vi "Measurement Logic.vi"() -> ()   [LabVIEW 2021, in "Line Transient Response_PMIC.lvlib"]
uses:
  Line Transient Response_PMIC.lvlib
  <vilib>/Plug-In SDKs/Measurements/Measure Call Context/Measure Call Context.lvclass
  Measurement Results.ctl
  Measurement Configuration.ctl
  <instrlib>/niDCPower/nidcpower.llb/niDCPower Source Mode.ctl
  <instrlib>/niDCPower/nidcpower.llb/niDCPower Wait For Event - Event.ctl
  <instrlib>/niScope/Controls/niScope trigger slope.ctl
  <instrlib>/niDCPower/nidcpower.llb/niDCPower Output Function.ctl
  <instrlib>/niDCPower/nidcpower.llb/niDCPower Aperture Time Units.ctl
  <instrlib>/niDCPower/nidcpower.llb/niDCPower Get Channel Name From String.vi
  <instrlib>/niScope/Utility/niScope Get Channel Name From String.vi
  <instrlib>/niScope/Configure/Trigger/niScope Configure Trigger Digital.vi
  <instrlib>/niDCPower/nidcpower.llb/niDCPower Configure Digital Edge Measure Trigger With Channels.vi
  <instrlib>/niDCPower/nidcpower.llb/niDCPower Configure Digital Edge Source Trigger With Channels.vi
  <instrlib>/niScope/Acquire/Fetch/niScope Fetch.vi
panel:
  in  "measurement configuration":T1={"DUT setup time"=1.0, "Nominal output voltage"=3.3, "Source resource name"="", "Source current limit"=0.25, "Source maximum power"=300.0, "Source sample rate"=1800000.0, "Source voltage set point 1"=7.0, "Source voltage set point 2"=20.0, "Source voltatge pulse duration"=0.005, "Source voltage delay t1"=0.005, "Source voltage delay t2"=0.005, "Source voltage falling slew rate"=50000.0, "Source voltage rising slew rate"=50000.0, "Source transient response"=1042, "Source voltage gain bandwidth"=2000.0, "Source voltage compensation frequency"=3530.0, "Source voltage pole-zero ratio"=2.0, "Load resource name"="", "Load voltage limit range"=4.0, "Load current level range"=4.0, "Load current level"=0.03, "Load transient response"=1042, "Load current gain bandwidth"=14000.0, "Load current compensation frequency"=180000.0, "Load current pole-zero ratio"=0.3, "Scope resource name"="", "Scope enable/disable"=TRUE, "Scope output channel name"="0", "Scope sample rate"=1800000.0, "Scope probe attenuation"=1.0, "Scope vertical range"=10.0, "Scope vertical coupling"=enum."DC", "Source Sense"=1008, "Load Sense"=1009, "Source update rate"=1000.0} {"Source update rate" format="%#_6pS/s"; "Load Sense" items=["Local"=1008, "Remote"=1009]; "Source Sense" items=["Local"=1008, "Remote"=1009]; "Source voltage delay t1" format="%#_8g"; "Scope vertical range" format="%.2f"; "Scope probe attenuation" format="%.1f"; "Scope sample rate" step=1000000.0 format="%#.2g"; "Load transient response" items=["Slow"=1041, "Normal"=1038, "Fast"=1039, "Custom"=1042]; "Source transient response" items=["Slow"=1041, "Normal"=1038, "Fast"=1039, "Custom"=1042]}
  out "measurement results":T2
  out "measure call context out":refnum<class "Measure Call Context.lvclass">
  in  "measure call context in":refnum<class "Measure Call Context.lvclass">
  out "error out":errorcluster
  in  "error in":errorcluster
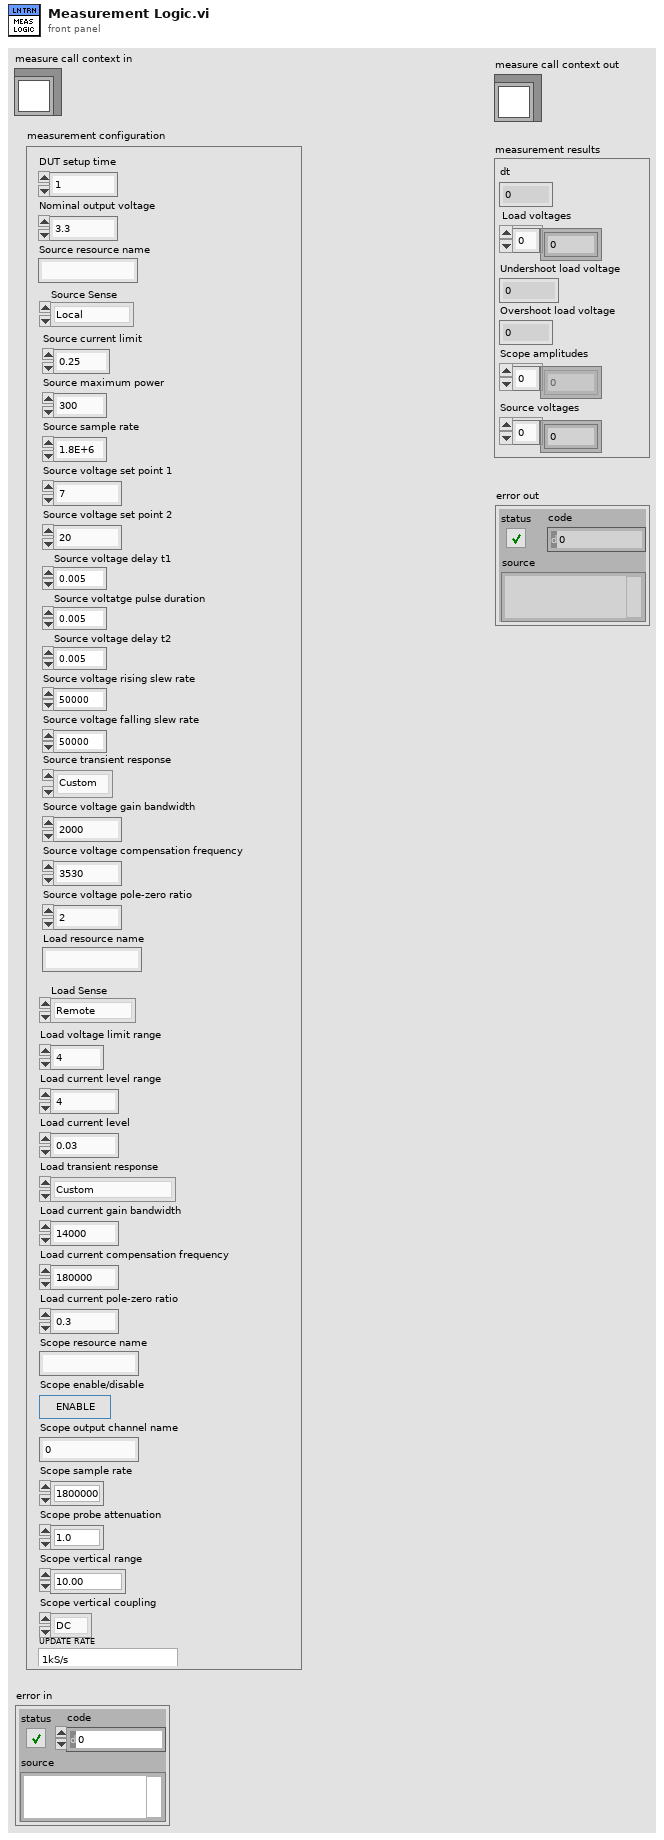
[diagram p1: front panel]
types:
  T1 = typedef "Line Transient Response_PMIC.lvlib/Measurement Configuration.ctl" = cluster{"DUT setup time":dbl, "Nominal output voltage":dbl, "Source resource name":string, "Source current limit":dbl, "Source maximum power":dbl, "Source sample rate":dbl, "Source voltage set point 1":dbl, "Source voltage set point 2":dbl, "Source voltatge pulse duration":dbl, "Source voltage delay t1":dbl, "Source voltage delay t2":dbl, "Source voltage falling slew rate":dbl, "Source voltage rising slew rate":dbl, "Source transient response":i32, "Source voltage gain bandwidth":dbl, "Source voltage compensation frequency":dbl, "Source voltage pole-zero ratio":dbl, "Load resource name":string, "Load voltage limit range":dbl, "Load current level range":dbl, "Load current level":dbl, "Load transient response":i32, "Load current gain bandwidth":dbl, "Load current compensation frequency":dbl, "Load current pole-zero ratio":dbl, "Scope resource name":string, "Scope enable/disable":bool, "Scope output channel name":string, "Scope sample rate":dbl, "Scope probe attenuation":dbl, "Scope vertical range":dbl, "Scope vertical coupling":enum32{"AC", "DC"}, "Source Sense":i32, "Load Sense":i32, "Source update rate":dbl}
  T2 = typedef "Line Transient Response_PMIC.lvlib/Measurement Results.ctl" = cluster{"dt":dbl, "Load voltages":dbl[], "Undershoot load voltage":dbl, "Overshoot load voltage":dbl, "Scope amplitudes":dbl[], "Source voltages":dbl[]}
  T3 = cluster{"Source out":refnum<k15>, "Source channel name":string, "Load out":refnum<k15>, "Load channel name":string, "Scope out":refnum<k15>, "Scope channel name":string, "Source sequence name":string, "Source terminal name":string, "Start source terminal name":string, "Measure load and scope terminal name":string, "Measure record length smu":i32, "Aperture time":dbl, "Measure record length scope":i32, "measurement results":T2}
  T4 = typedef "niDCPower Wait For Event - Event.ctl" = i32
  T5 = typedef "niDCPower Source Mode.ctl" = i32
  T6 = typedef "niScope trigger slope.ctl" = i32
  T7 = typedef "niDCPower Aperture Time Units.ctl" = i32
  T8 = typedef "niDCPower Output Function.ctl" = i32
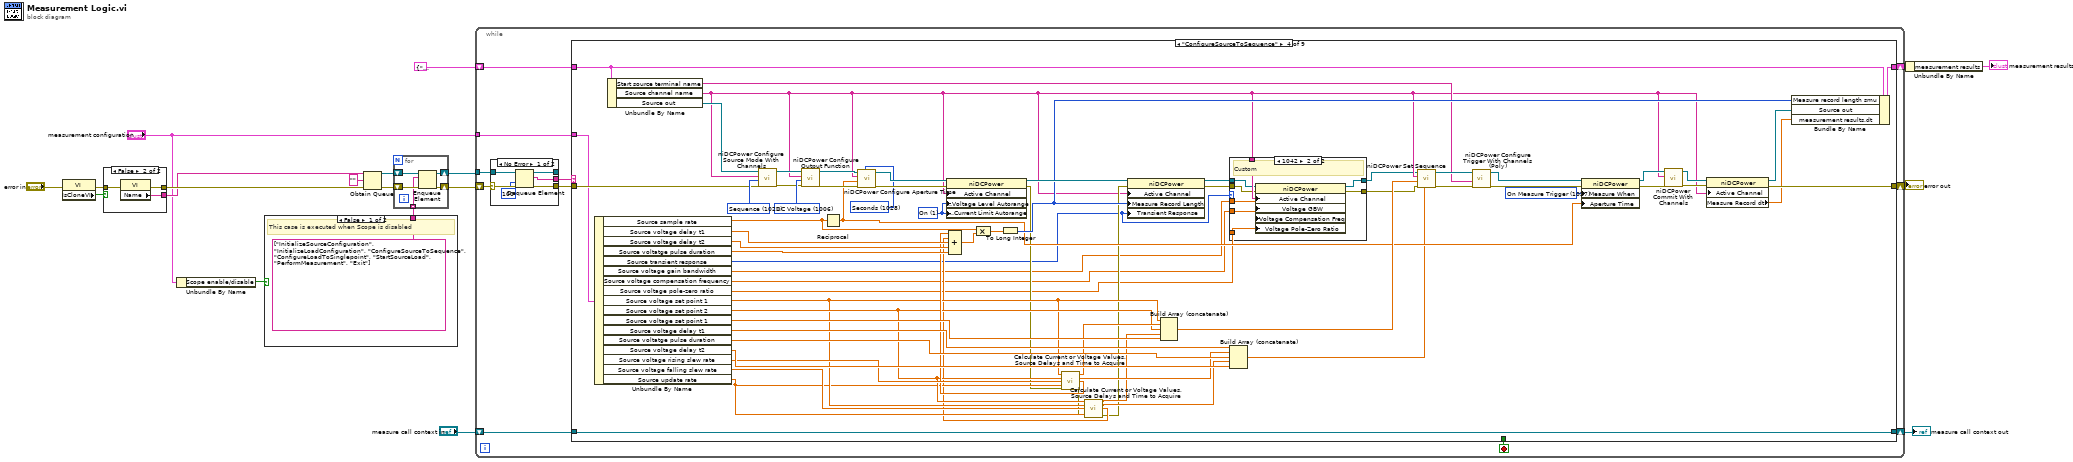
[diagram p0: block diagram]
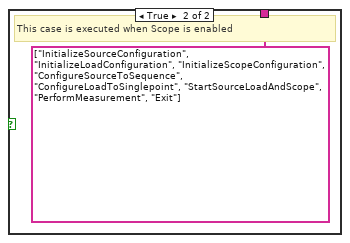
[diagram p2: hidden frame]
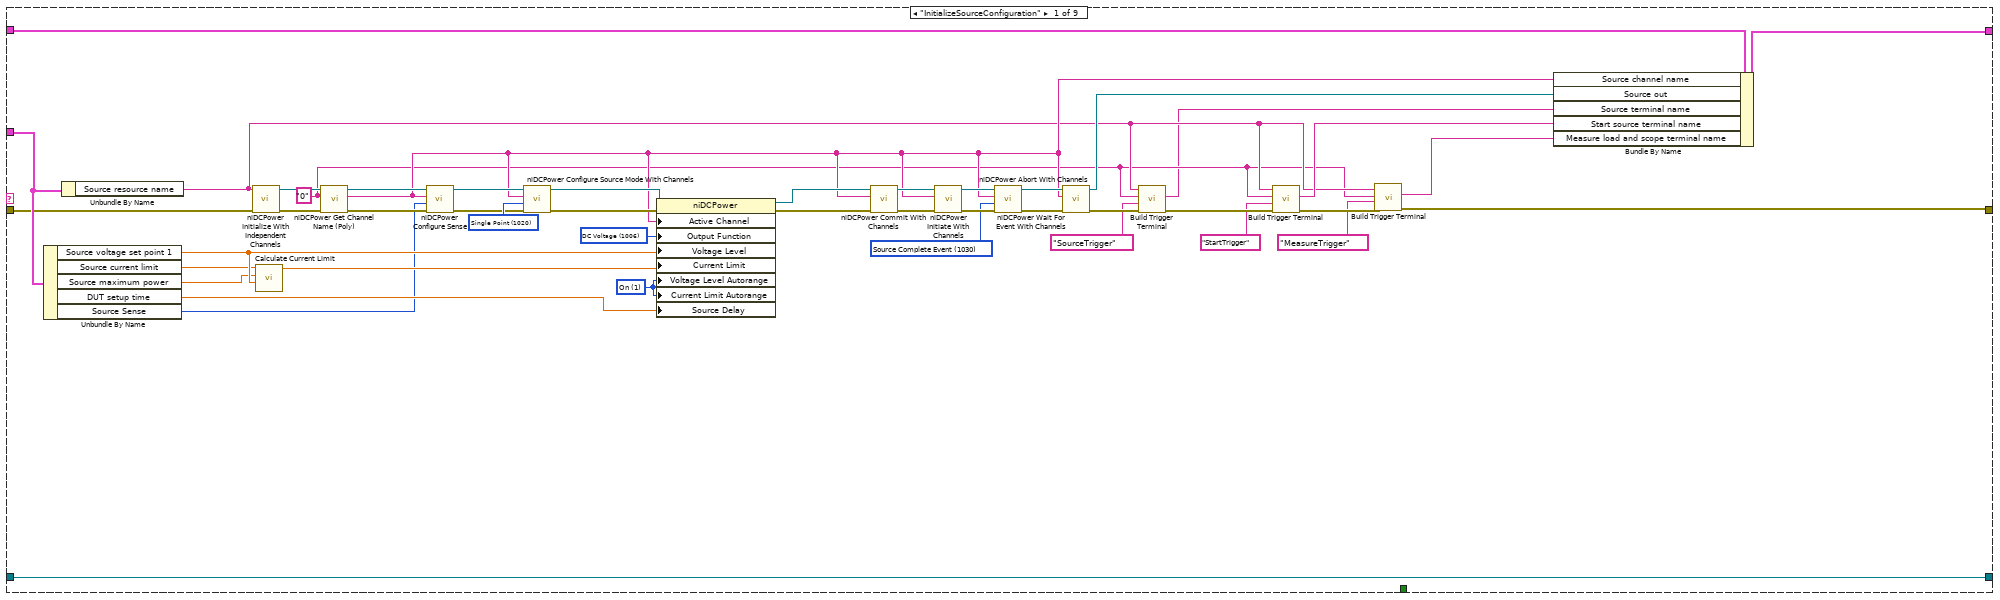
[diagram p3: hidden frame]
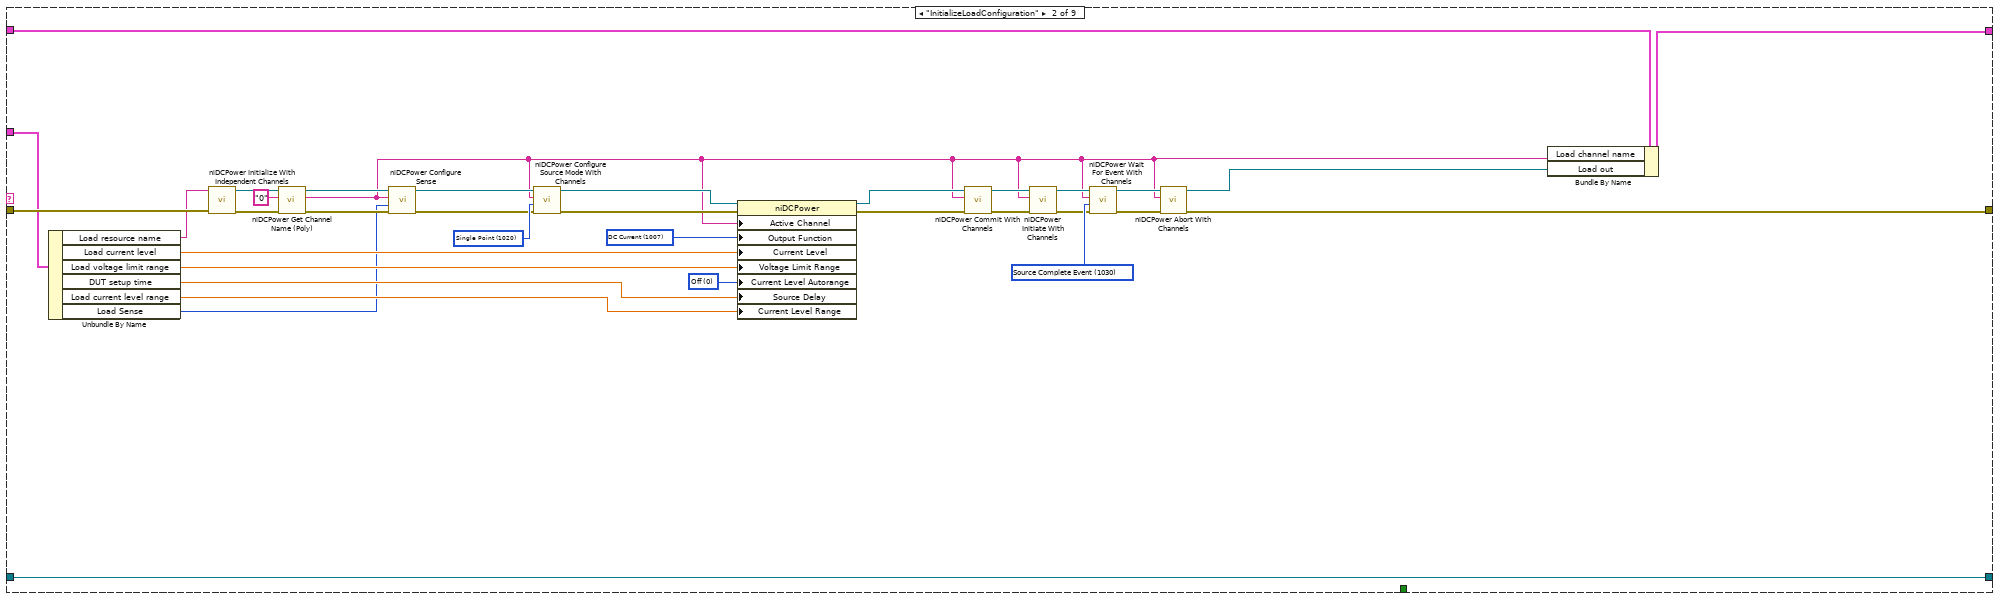
[diagram p4: hidden frame]
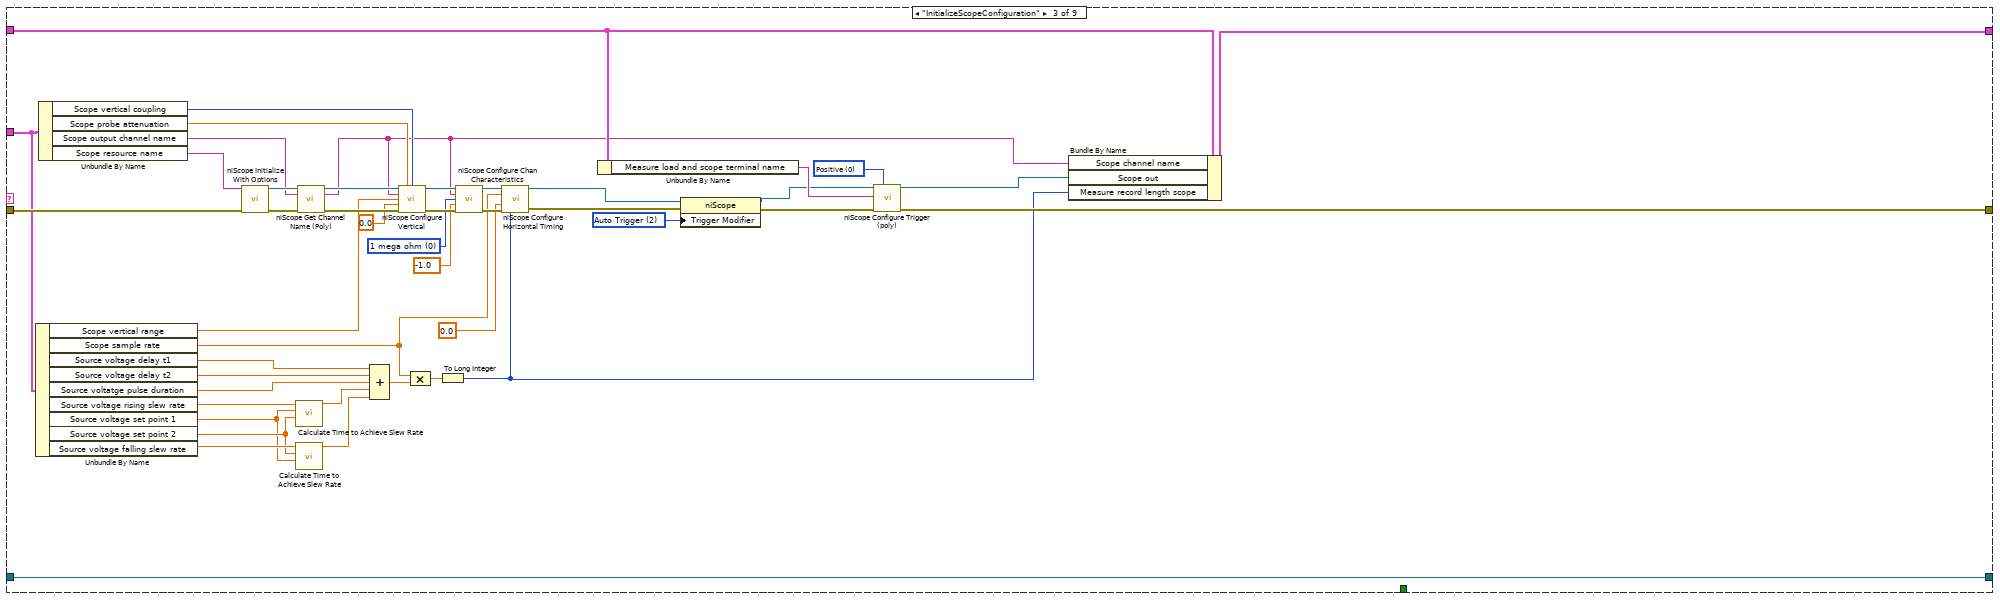
[diagram p5: hidden frame]
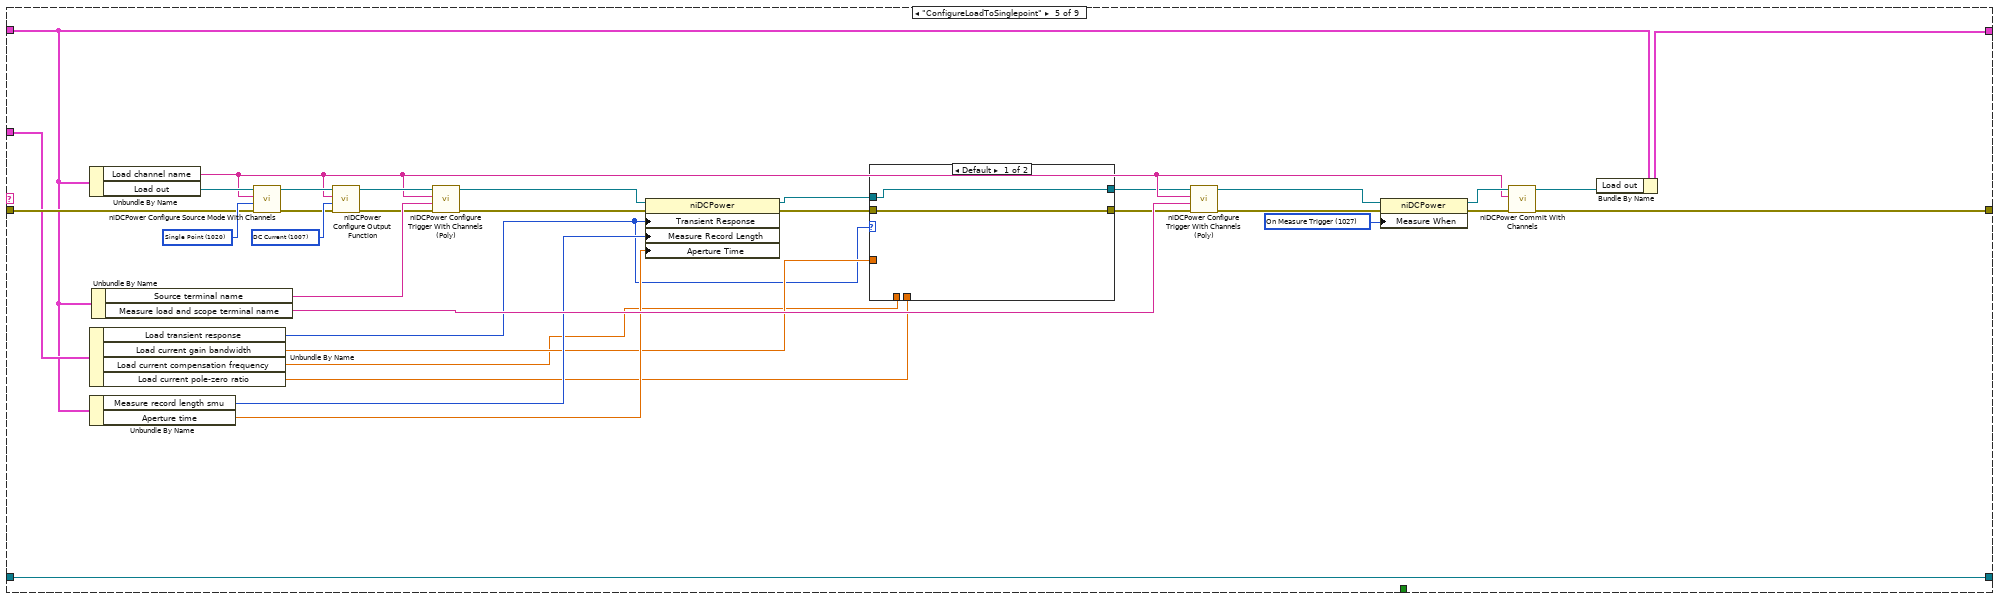
[diagram p7: hidden frame]
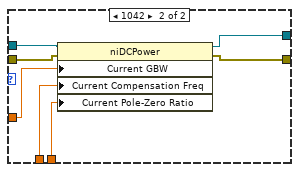
[diagram p8: hidden frame]
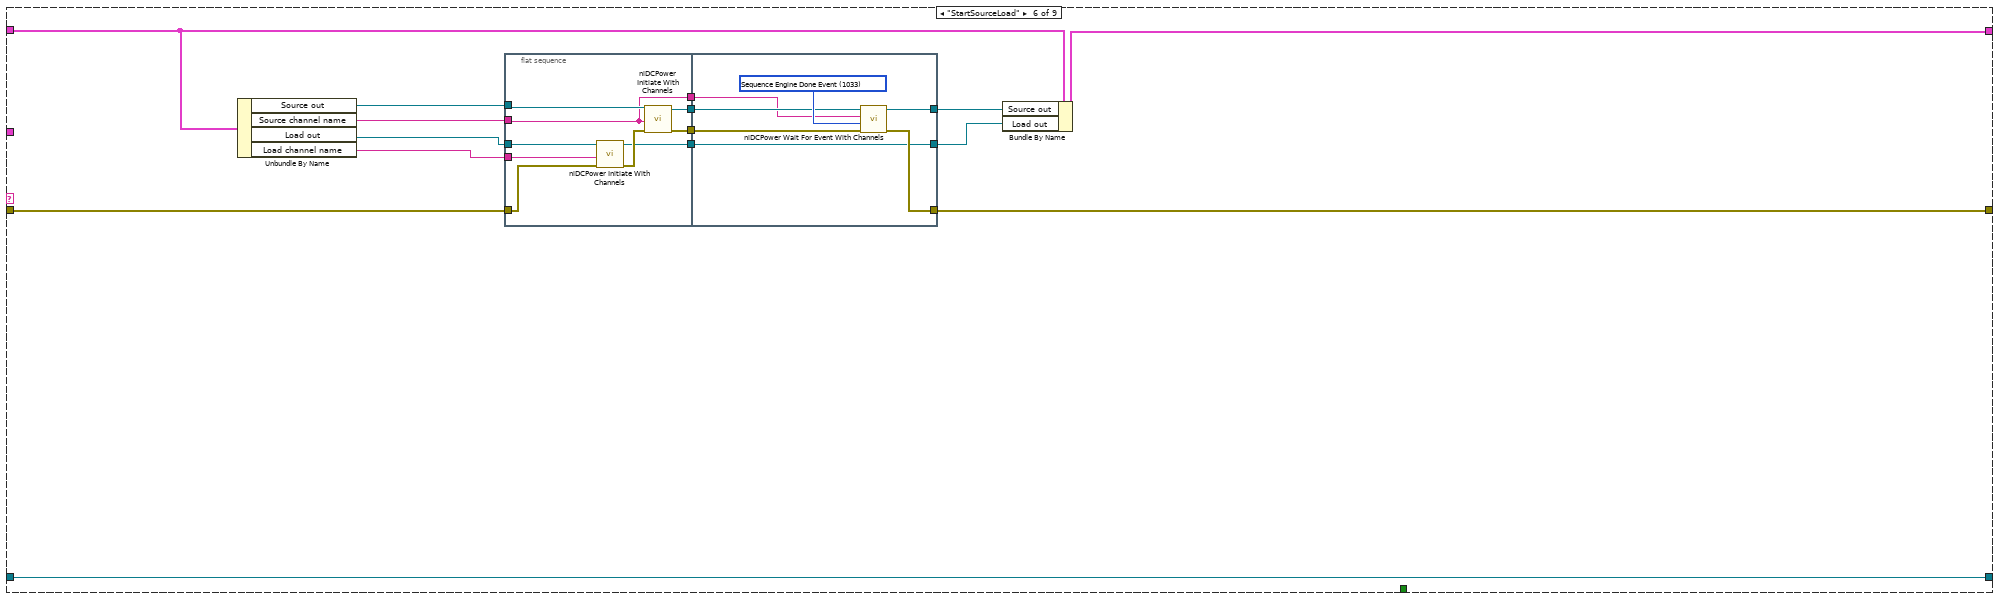
[diagram p9: hidden frame]
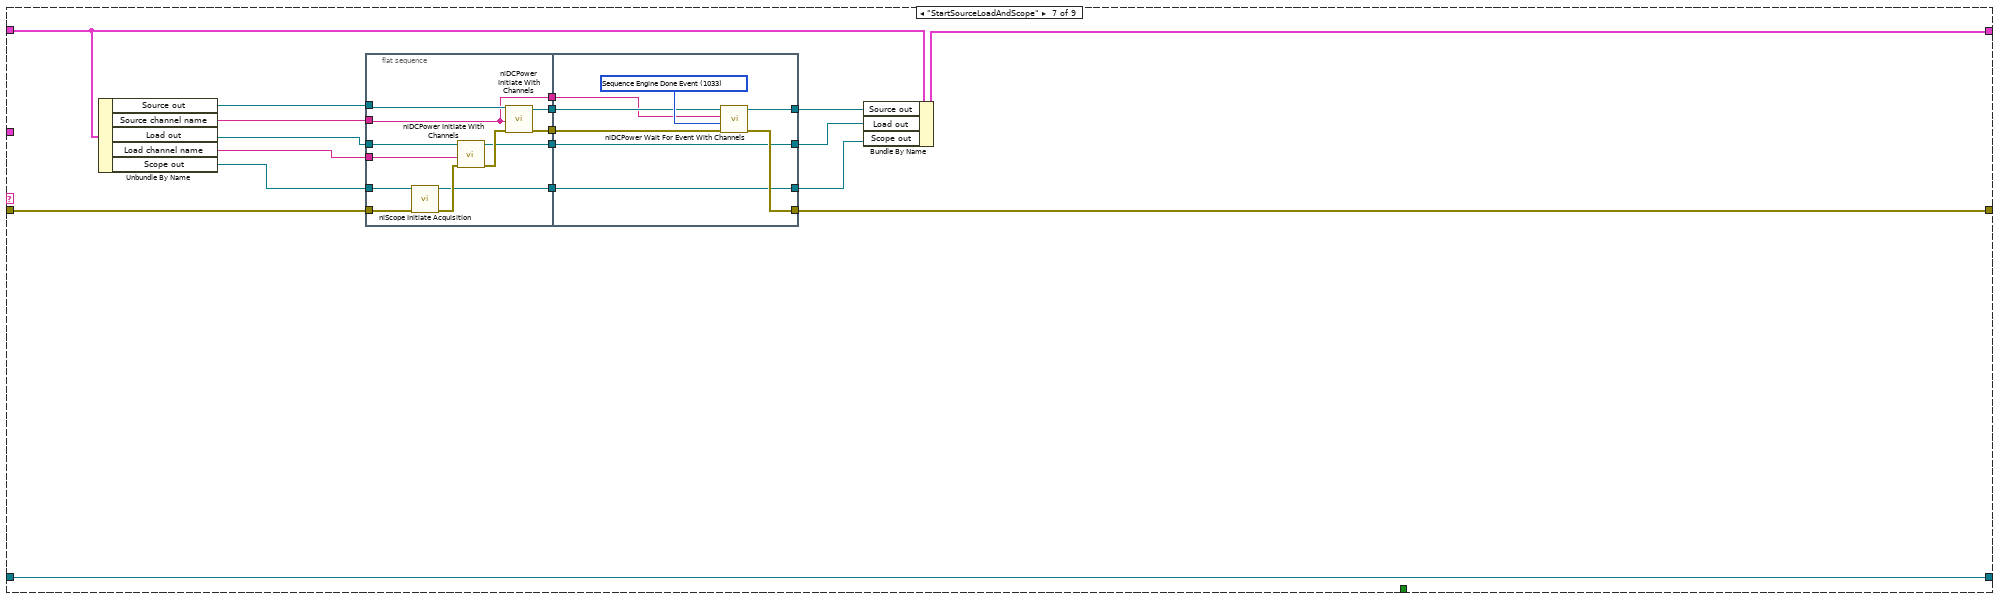
[diagram p10: hidden frame]
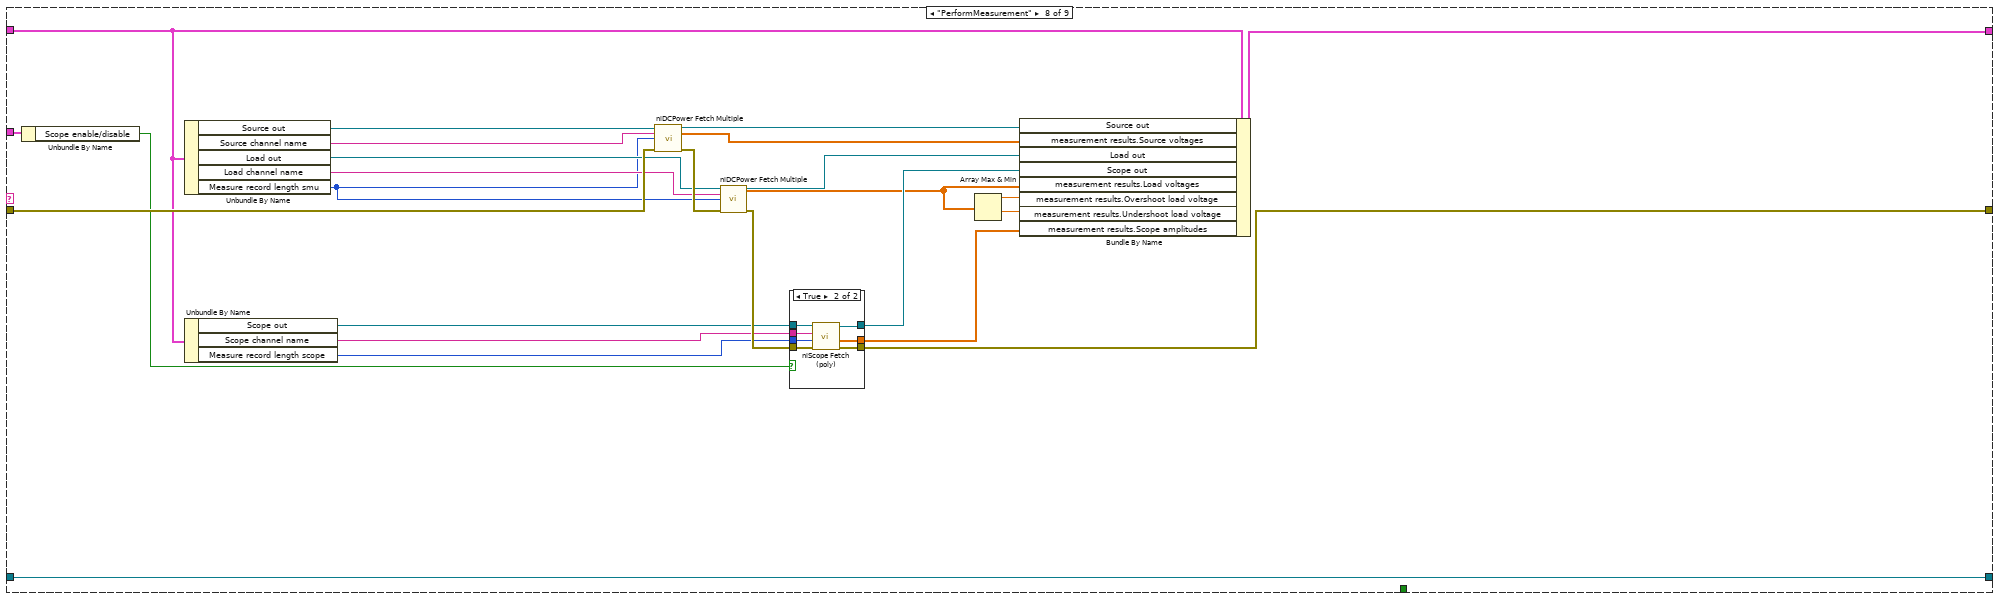
[diagram p11: hidden frame]
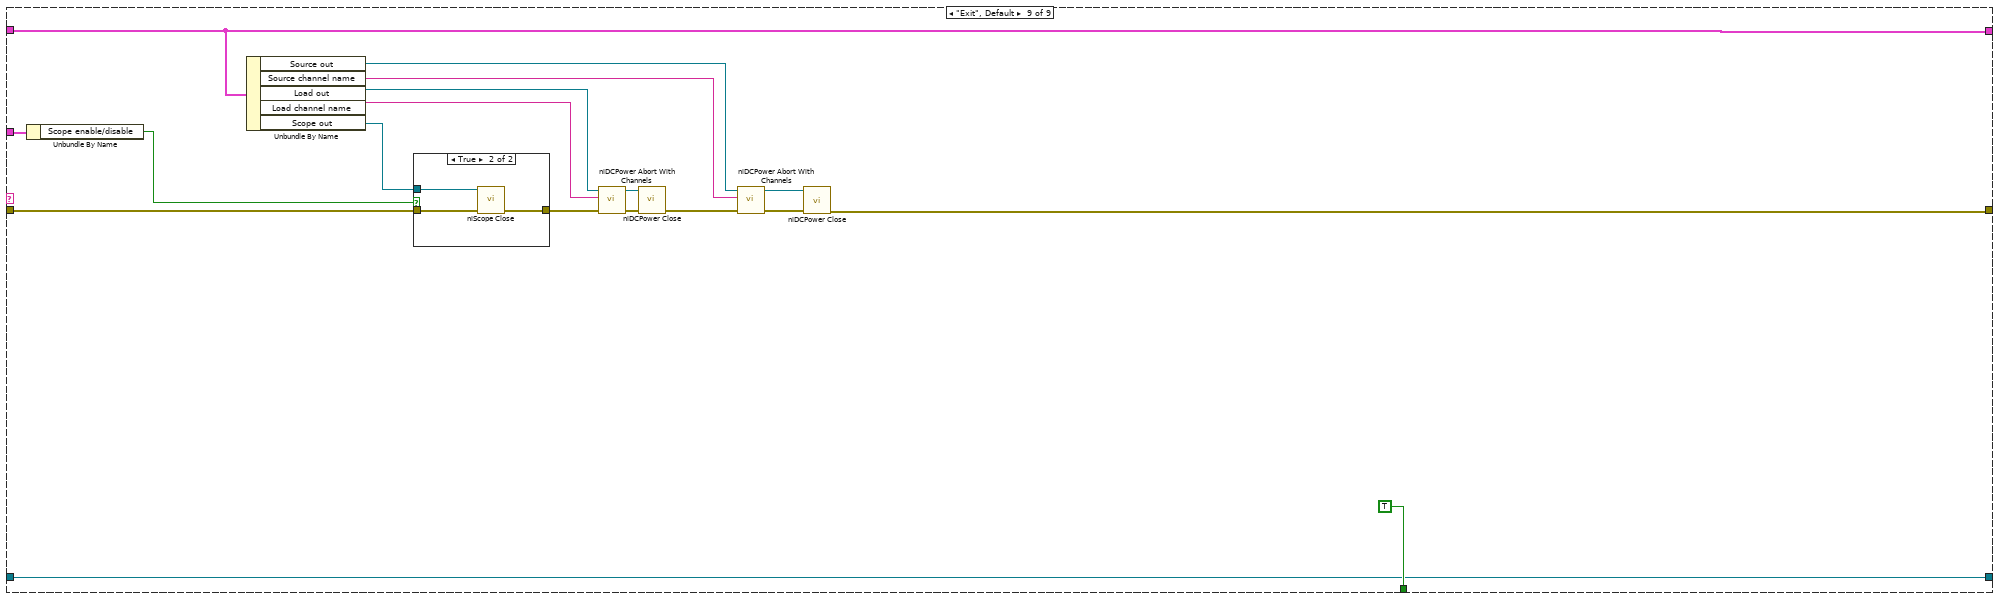
[diagram p13: hidden frame]
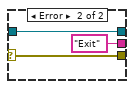
[diagram p15: hidden frame]
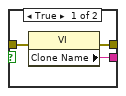
[diagram p16: hidden frame]
diagram:
  n1 = property class="VI"(error in="error in") -> (error out=w18:errorcluster, "IsCloneVI"=w19:bool)  [unwired: 1 in, 1 out]
  n2 = case shown="False" w19 {
    tunnel: [w22 w25] -> w17
    tunnel: [w21 w24] -> w16
    tunnel: w18 -> [w20 w23]
    frame True {
      n3 = property class="VI"(error in=w20) -> (error out=w22:errorcluster, "Clone Name"=w21:string)  [unwired: 1 in, 1 out]
    }
    frame False {
      n4 = property class="VI"(error in=w23) -> (error out=w25:errorcluster, "Name"=w24:string)  [unwired: 1 in, 1 out]
    }
  }
  n5 = Unbundle By Name("measurement configuration") -> ("Scope enable/disable"=w3:bool)
  n6 = case shown="False" w3 {
    tunnel: [string[] ["InitializeSourceConfiguration", "InitializeLoadConfiguration", "ConfigureSourceToSequence", "ConfigureLoadToSinglepoint", "StartSourceLoad", "PerformMeasurement", "Exit"] ("Step sequence") string[] ["InitializeSourceConfiguration", "InitializeLoadConfiguration", "InitializeScopeConfiguration", "ConfigureSourceToSequence", "ConfigureLoadToSinglepoint", "StartSourceLoadAndScope", "PerformMeasurement", "Exit"] ("Step sequence")] -> w12
    frame False {
      # "This case is executed when Scope is disabled"
    }
    frame True {
      # "This case is executed when Scope is enabled"
    }
  }
  n7 = Obtain Queue(name (unnamed)=w16, element data type="", error in (no error)=w17) -> (queue out=w14:refnum<queue>, error out=w15:errorcluster)  [unwired: 2 in, 1 out]
  n8 = for {
    shift-right: [w30] -> w11
    shift-left: w14 -> [w32]
    shift-right: [w29] -> w10
    shift-left: w15 -> [w31]
    tunnel: w12 -> [w28] mode=indexing
    n9 = Enqueue Element(queue=w32, element=w28, error in (no error)=w31) -> (queue out=w30:refnum<queue>, error out=w29:errorcluster)  [unwired: 1 in, 1 out]
  }
  n10 = while {
    tunnel: w11 -> [w43]
    shift-right: [w36] -> w8
    shift-left: w10 -> [w42]
    tunnel: "measurement configuration" -> [w40]
    shift-right: [w38] -> w7
    shift-left: T3 {"Source out"="", "Source channel name"="", "Load out"="", "Load channel name"="", "Scope out"="", "Scope channel name"="", "Source sequence name"="", "Source terminal name"="", "Start source terminal name"="", "Measure load and scope terminal name"="", "Measure record length smu"=0, "Aperture time"=0.0, "Measure record length scope"=0, "measurement results"={"dt"=0.0, "Load voltages"=[0.0], "Undershoot load voltage"=0.0, "Overshoot load voltage"=0.0, "Scope amplitudes"=[], "Source voltages"=[0.0]}} -> [w39]
    shift-right: [w34] -> w5
    shift-left: "measure call context in" -> [w33]
    stop <- w35 stop-if-true
    n11 = case shown="No Error" w42 {
      selector: w42 -> [w417 w421]
      tunnel: w43 -> [w419 w420]
      tunnel: [w418 "Exit" ("t")] -> w41
      tunnel: [w416 w421] -> w37
      tunnel: [w414 w420] -> _
      frame No Error {
        n12 = Dequeue Element(queue=w419, timeout in ms (-1)=100, error in (no error)=w417) -> (queue out=w414:refnum<queue>, element=w418:string, error out=w416:errorcluster)  [unwired: 1 out]
      }
      frame Error {
      }
    }
    n13 = case shown="\"ConfigureSourceToSequence\"" w41 {
      tunnel: w40 -> [w66 w97 w152 w214 w267 _ _ w377 w404]
      tunnel: w39 -> [w65 w95 w145 w213 w263 w292 w329 w381 w405]
      tunnel: [w64 w96 w144 w212 w261 w291 w323 w380 w405] -> w38
      tunnel: w37 -> [w63 w99 w153 w215 w268 w293 w328 w382 w409]
      tunnel: [w49 w93 w147 w211 w264 w290 w324 w379 w408] -> w36
      tunnel: [_ _ _ _ _ _ _ _ TRUE] -> w35
      tunnel: [w62 w94 w141 w210 w260 w289 w320 w378 w406] -> w34
      tunnel: w33 -> [w62 w94 w141 w210 w260 w289 w320 w378 w406]
      frame "InitializeSourceConfiguration" {
        w47 = "0" ("index")
        w72 = 1 items=["Off", "On"] ("Source:DC Voltage:Voltage Level Autorange")
        w73 = T4 1030 items=["Source Complete Event"=1030, "Measure Complete Event"=1031, "Sequence Iteration Complete Event"=1032, "Sequence Engine Done Event"=1033, "Pulse Complete Event"=1051, "Ready For Pulse Trigger Event"=1052] ("event")
        w84 = T5 1020 items=["Single Point"=1020, "Sequence"=1021] ("source mode")
        w79 = 1006 items=["DC Voltage"=1006, "DC Current"=1007, "Pulse Voltage"=1049, "Pulse Current"=1050] ("Source:Output Function")
        n14 = Unbundle By Name(w66) -> ("Source voltage set point 1"=w57:dbl, "Source current limit"=w54:dbl, "Source maximum power"=w55:dbl, "DUT setup time"=w58:dbl, "Source Sense"=w44:i32)
        n15 = Unbundle By Name(w66) -> ("Source resource name"=w48:string)
        n16 = call <instrlib>:"niDCPower Initialize With Independent Channels.vi"("error in (no error)"=w63, "resource name"=w48) -> ("error out"=w70:errorcluster, "instrument handle out"=w74:refnum<k15>)  [unwired: 8 in]
        n17 = call "Calculate Current Limit.vi"("Voltage value"=w57, "Maximum power"=w55, "Current limit in"=w54) -> ("Current limit out"=w56:dbl)  [unwired: 8 in]
        n18 = call-poly <instrlib>:"niDCPower Get Channel Name (Poly).vi"("error in (no error)"=w70, "index"=w47, "instrument handle"=w74) -> ("error out"=w69:errorcluster, "name"=w68:string, "instrument handle out"=w71:refnum<k15>)  [unwired: 6 in]
        n19 = call <instrlib>:"niDCPower Configure Sense.vi"("error in (no error)"=w69, "sense"=w44, "channel name"=w68, "instrument handle"=w71) -> ("error out"=w82:errorcluster, "instrument handle out"=w80:refnum<k15>)  [unwired: 6 in]
        n20 = call <instrlib>:"niDCPower Configure Source Mode With Channels.vi"("error in (no error)"=w82, "source mode"=w84, "channel name"=w68, "instrument handle"=w80) -> ("error out"=w83:errorcluster, "instrument handle out"=w81:refnum<k15>)  [unwired: 6 in]
        n21 = property class="niDCPower"(reference=w81, error in=w83, "Active Channel"=w68, "Output Function"=w79, "Voltage Level"=w57, "Current Limit"=w56, "Voltage Level Autorange"=w72, "Current Limit Autorange"=w72, "Source Delay"=w58) -> (reference out=w85:refnum<k15>, error out=w86:errorcluster)
        n22 = call <instrlib>:"niDCPower Commit With Channels.vi"("error in (no error)"=w86, "channel name"=w68, "instrument handle"=w85) -> ("error out"=w88:errorcluster, "instrument handle out"=w87:refnum<k15>)  [unwired: 7 in]
        n23 = call <instrlib>:"niDCPower Initiate With Channels.vi"("error in (no error)"=w88, "channel name"=w68, "instrument handle"=w87) -> ("error out"=w75:errorcluster, "instrument handle out"=w76:refnum<k15>)  [unwired: 7 in]
        n24 = call <instrlib>:"niDCPower Wait For Event With Channels.vi"("error in (no error)"=w75, "event"=w73, "channel name"=w68, "instrument handle"=w76) -> ("error out"=w78:errorcluster, "instrument handle out"=w77:refnum<k15>)  [unwired: 6 in]
        n25 = call <instrlib>:"niDCPower Abort With Channels.vi"("error in (no error)"=w78, "channel name"=w68, "instrument handle"=w77) -> ("error out"=w61:errorcluster, "instrument handle out"=w67:refnum<k15>)  [unwired: 7 in]
        n26 = call "Build Trigger Terminal.vi"("error in (no error)"=w61, "Trigger/Event Name"="SourceTrigger", "Channel Name"=w47, "Resource Name"=w48) -> ("error out"=w59:errorcluster, "Terminal Name"=w45:string)  [unwired: 6 in]
        n27 = call "Build Trigger Terminal.vi"("error in (no error)"=w59, "Trigger/Event Name"="StartTrigger", "Channel Name"=w47, "Resource Name"=w48) -> ("error out"=w51:errorcluster, "Terminal Name"=w52:string)  [unwired: 6 in]
        n28 = call "Build Trigger Terminal.vi"("error in (no error)"=w51, "Trigger/Event Name"="MeasureTrigger", "Channel Name"=w47, "Resource Name"=w48) -> ("error out"=w49:errorcluster, "Terminal Name"=w46:string)  [unwired: 6 in]
        n29 = Bundle By Name(cluster=w65, "Source channel name"=w68, "Source out"=w67, "Source terminal name"=w45, "Start source terminal name"=w52, "Measure load and scope terminal name"=w46) -> (w64:T3)
      }
      frame "InitializeLoadConfiguration" {
        w119 = T5 1020 items=["Single Point"=1020, "Sequence"=1021] ("source mode")
        w112 = T4 1030 items=["Source Complete Event"=1030, "Measure Complete Event"=1031, "Sequence Iteration Complete Event"=1032, "Sequence Engine Done Event"=1033, "Pulse Complete Event"=1051, "Ready For Pulse Trigger Event"=1052] ("event")
        w107 = 0 items=["Off", "On"] ("Source:DC Current:Current Level Autorange")
        w108 = 1007 items=["DC Voltage"=1006, "DC Current"=1007, "Pulse Voltage"=1049, "Pulse Current"=1050] ("Source:Output Function")
        n30 = Unbundle By Name(w97) -> ("Load resource name"=w92:string, "Load current level"=w101:dbl, "Load voltage limit range"=w100:dbl, "DUT setup time"=w106:dbl, "Load current level range"=w98:dbl, "Load Sense"=w89:i32)
        n31 = call <instrlib>:"niDCPower Initialize With Independent Channels.vi"("error in (no error)"=w99, "resource name"=w92) -> ("error out"=w104:errorcluster, "instrument handle out"=w109:refnum<k15>)  [unwired: 8 in]
        n32 = call-poly <instrlib>:"niDCPower Get Channel Name (Poly).vi"("error in (no error)"=w104, "index"="0", "instrument handle"=w109) -> ("error out"=w103:errorcluster, "name"=w90:string, "instrument handle out"=w105:refnum<k15>)  [unwired: 6 in]
        n33 = call <instrlib>:"niDCPower Configure Sense.vi"("error in (no error)"=w103, "sense"=w89, "channel name"=w90, "instrument handle"=w105) -> ("error out"=w116:errorcluster, "instrument handle out"=w115:refnum<k15>)  [unwired: 6 in]
        n34 = call <instrlib>:"niDCPower Configure Source Mode With Channels.vi"("error in (no error)"=w116, "source mode"=w119, "channel name"=w90, "instrument handle"=w115) -> ("error out"=w118:errorcluster, "instrument handle out"=w117:refnum<k15>)  [unwired: 6 in]
        n35 = property class="niDCPower"(reference=w117, error in=w118, "Active Channel"=w90, "Output Function"=w108, "Current Level"=w101, "Voltage Limit Range"=w100, "Current Level Autorange"=w107, "Source Delay"=w106, "Current Level Range"=w98) -> (reference out=w120:refnum<k15>, error out=w121:errorcluster)
        n36 = call <instrlib>:"niDCPower Commit With Channels.vi"("error in (no error)"=w121, "channel name"=w90, "instrument handle"=w120) -> ("error out"=w122:errorcluster, "instrument handle out"=w123:refnum<k15>)  [unwired: 7 in]
        n37 = call <instrlib>:"niDCPower Initiate With Channels.vi"("error in (no error)"=w122, "channel name"=w90, "instrument handle"=w123) -> ("error out"=w110:errorcluster, "instrument handle out"=w111:refnum<k15>)  [unwired: 7 in]
        n38 = call <instrlib>:"niDCPower Wait For Event With Channels.vi"("error in (no error)"=w110, "event"=w112, "channel name"=w90, "instrument handle"=w111) -> ("error out"=w114:errorcluster, "instrument handle out"=w113:refnum<k15>)  [unwired: 6 in]
        n39 = call <instrlib>:"niDCPower Abort With Channels.vi"("error in (no error)"=w114, "channel name"=w90, "instrument handle"=w113) -> ("error out"=w93:errorcluster, "instrument handle out"=w102:refnum<k15>)  [unwired: 7 in]
        n40 = Bundle By Name(cluster=w95, "Load channel name"=w90, "Load out"=w102) -> (w96:T3)
      }
      frame "InitializeScopeConfiguration" {
        w157 = 2 items=["None"=1, "Auto Trigger"=2] ("Trigger Modifier")
        w139 = u32 0 items=["1 mega ohm"=0, "50 ohms"=2] ("Input Impedance")
        w154 = T6 0 items=["Positive", "Negative"] ("trigger slope")
        n41 = Unbundle By Name(w152) -> ("Scope vertical range"=w138:dbl, "Scope sample rate"=w148:dbl, "Source voltage delay t1"=w136:dbl, "Source voltage delay t2"=w135:dbl, "Source voltatge pulse duration"=w134:dbl, "Source voltage rising slew rate"=w132:dbl, "Source voltage set point 1"=w127:dbl, "Source voltage set point 2"=w128:dbl, "Source voltage falling slew rate"=w130:dbl)
        n42 = Unbundle By Name(w152) -> ("Scope vertical coupling"=w149:enum32{"AC", "DC"}, "Scope probe attenuation"=w150:dbl, "Scope output channel name"=w140:string, "Scope resource name"=w151:string)
        n43 = call <instrlib>:"niScope Initialize With Options.vi"("resource name"=w151, "error in"=w153) -> ("instrument handle"=w168:refnum<k15>, "error out"=w167:errorcluster)  [unwired: 12 in]
        n44 = call "Calculate Time to Achieve Slew Rate.vi"("Current/voltage set point 2"=w128, "Current/voltage set point 1"=w127, "Current/voltage slew rate"=w132) -> ("Calculated time"=w131:dbl)  [unwired: 8 in]
        n45 = call "Calculate Time to Achieve Slew Rate.vi"("Current/voltage set point 2"=w127, "Current/voltage set point 1"=w128, "Current/voltage slew rate"=w130) -> ("Calculated time"=w129:dbl)  [unwired: 8 in]
        n46 = call-poly <instrlib>:"niScope Get Channel Name (Poly).vi"("instrument handle"=w168, "index"=w140, "error in"=w167) -> ("instrument handle out"=w156:refnum<k15>, "channel name"=w142:string, "error out"=w155:errorcluster)  [unwired: 10 in]
        n47 = Compound Arithmetic op=ADD(w136, w135, w134, w131, w129) -> (w124:dbl)
        n48 = call <instrlib>:"niScope Configure Vertical.vi"("instrument handle"=w156, "probe attenuation"=w150, "vertical coupling"=w149, "channels"=w142, "vertical range"=w138, "vertical offset"=0.0, "error in"=w155) -> ("instrument handle out"=w166:refnum<k15>, "error out"=w165:errorcluster)  [unwired: 7 in]
        n49 = Compound Arithmetic op=MULTIPLY(w148, w124) -> (w126:dbl)
        n50 = To Long Integer(number=w126) -> (32bit integer=w125:i32)
        n51 = call <instrlib>:"niScope Configure Chan Characteristics.vi"("instrument handle"=w166, "channels"=w142, "input impedance"=w139, "maximum input frequency"=-1.0 ("Maximum Input Frequency"), "error in"=w165) -> ("instrument handle out"=w163:refnum<k15>, "error out"=w164:errorcluster)  [unwired: 9 in]
        n52 = call <instrlib>:"niScope Configure Horizontal Timing.vi"("instrument handle"=w163, "min sample rate"=w148, "reference position"=0.0 ("Reference Position"), "error in"=w164, "min record length"=w125) -> ("instrument handle out"=w160:refnum<k15>, "error out"=w159:errorcluster)  [unwired: 9 in]
        n53 = Unbundle By Name(w145) -> ("Measure load and scope terminal name"=w146:string)
        n54 = property on="Property Node" class="niScope"(reference=w160, error in=w159, "Trigger Modifier"=w157) -> (reference out=w133:refnum<k15>, error out=w158:errorcluster)
        n55 = call-poly <instrlib>:"niScope Configure Trigger (poly).vi"("instrument handle"=w133, "trigger slope"=w154, "trigger source"=w146, "error in"=w158) -> ("instrument handle out"=w143:refnum<k15>, "error out"=w147:errorcluster)  [unwired: 10 in]
        n56 = Bundle By Name(cluster=w145, "Scope channel name"=w142, "Scope out"=w143, "Measure record length scope"=w125) -> (w144:T3)
      }
      frame "ConfigureSourceToSequence" {
        w221 = T7 1028 items=["Seconds"=1028, "Powerline Cycles"=1029] ("aperture time units")
        w228 = 1027 items=["Automatically after Source Complete"=1025, "On Demand"=1026, "On Measure Trigger"=1027] ("Measurement:Advanced:Measure When")
        w233 = 1 items=["Off", "On"] ("DC Voltage:Voltage Level Autorange")
        w232 = T8 1006 items=["DC Voltage"=1006, "DC Current"=1007, "Pulse Voltage"=1049, "Pulse Current"=1050] ("output function")
        w231 = T5 1021 items=["Single Point"=1020, "Sequence"=1021] ("source mode")
        n57 = Unbundle By Name(w214) -> ("Source sample rate"=w195:dbl, "Source voltage delay t1"=w208:dbl, "Source voltage delay t2"=w194:dbl, "Source voltatge pulse duration"=w206:dbl, "Source transient response"=w173:i32, "Source voltage gain bandwidth"=w177:dbl, "Source voltage compensation frequency"=w176:dbl, "Source voltage pole-zero ratio"=w175:dbl, "Source voltage set point 1"=w186:dbl, "Source voltage set point 2"=w187:dbl, "Source voltage set point 1"=w192:dbl, "Source voltage delay t1"=w199:dbl, "Source voltatge pulse duration"=w197:dbl, "Source voltage delay t2"=w196:dbl, "Source voltage rising slew rate"=w191:dbl, "Source voltage falling slew rate"=w185:dbl, "Source update rate"=w184:dbl)
        n58 = Unbundle By Name(w213) -> ("Start source terminal name"=w200:string, "Source channel name"=w174:string, "Source out"=w235:refnum<k15>)
        n59 = call <instrlib>:"niDCPower Configure Source Mode With Channels.vi"("error in (no error)"=w215, "source mode"=w231, "channel name"=w174, "instrument handle"=w235) -> ("error out"=w229:errorcluster, "instrument handle out"=w230:refnum<k15>)  [unwired: 6 in]
        n60 = call <instrlib>:"niDCPower Configure Output Function.vi"("error in (no error)"=w229, "output function"=w232, "channel name"=w174, "instrument handle"=w230) -> ("error out"=w225:errorcluster, "instrument handle out"=w223:refnum<k15>)  [unwired: 6 out]
        n61 = Reciprocal(x=w195) -> (1/x=w205:dbl)
        n62 = call <instrlib>:"niDCPower Configure Aperture Time.vi"("aperture time units"=w221, "error in (no error)"=w225, "aperture time"=w205, "channel name"=w174, "instrument handle"=w223) -> ("error out"=w224:errorcluster, "instrument handle out"=w222:refnum<k15>)  [unwired: 5 in]
        n63 = property class="niDCPower"(reference=w222, error in=w224, "Active Channel"=w174, "Source:DC Voltage:Voltage Level Autorange"=w233, "Source:DC Voltage:Current Limit Autorange"=w233) -> (reference out=w234:refnum<k15>, error out=w179:errorcluster)
        n64 = call "Calculate Current or Voltage Values, Source Delays and Time to Acquire.vi"("Current/voltage start point (AorV)"=w186, "Current/voltage end point (AorV)"=w187, "Current/voltage slew rate (AorV/sec)"=w191, "Update Rate (S/sec)"=w184, "error in (no error)"=w179) -> ("Current or voltage values"=w190:dbl[], "Source delays (sec)"=w189:dbl[], "Time to acquire (sec)"=w188:dbl, "error out"=w180:errorcluster)  [unwired: 6 in, 1 out]
        n65 = call "Calculate Current or Voltage Values, Source Delays and Time to Acquire.vi"("Current/voltage start point (AorV)"=w187, "Current/voltage end point (AorV)"=w186, "Current/voltage slew rate (AorV/sec)"=w185, "Update Rate (S/sec)"=w184, "error in (no error)"=w180) -> ("Current or voltage values"=w183:dbl[], "Source delays (sec)"=w182:dbl[], "Time to acquire (sec)"=w181:dbl, "error out"=w178:errorcluster)  [unwired: 6 in, 1 out]
        n66 = Compound Arithmetic op=ADD(w188, w181, w208, w194, w206) -> (w207:dbl)
        n67 = Compound Arithmetic op=MULTIPLY(w195, w207) -> (w220:dbl)
        n68 = To Long Integer(number=w220) -> (32bit integer=w209:i32)
        n69 = property class="niDCPower"(reference=w234, error in=w178, "Active Channel"=w174, "Measure Record Length"=w209, "Transient Response"=w173) -> (reference out=w172:refnum<k15>, error out=w171:errorcluster)
        n70 = Build Array (concatenate)(w186, w190, w187, w183, w192) -> (w219:dbl[])
        n71 = case shown="1042" w173 {
          tunnel: w177 -> [_ w245]
          tunnel: w176 -> [_ w244]
          tunnel: w175 -> [_ w243]
          tunnel: w174 -> [_ w242]
          tunnel: w172 -> [w237 w241]
          tunnel: w171 -> [w236 w240]
          tunnel: [w237 w239] -> w170
          tunnel: [w236 w238] -> w169
          frame Default {
            # "fast,slow,normal"
          }
          frame 1042 {
            # "Custom"
            n72 = property class="niDCPower"(reference=w241, error in=w240, "Active Channel"=w242, "Voltage GBW"=w245, "Voltage Compensation Freq"=w244, "Voltage Pole-Zero Ratio"=w243) -> (reference out=w239:refnum<k15>, error out=w238:errorcluster)
          }
        }
        n73 = Build Array (concatenate)(w199, w189, w197, w182, w196) -> (w198:dbl[])
        n74 = call <instrlib>:"niDCPower Set Sequence.vi"("source delays"=w198, "error in (no error)"=w169, "values"=w219, "channel name"=w174, "instrument handle"=w170) -> ("error out"=w203:errorcluster, "instrument handle out"=w204:refnum<k15>)  [unwired: 5 in]
        n75 = call-poly <instrlib>:"niDCPower Configure Trigger With Channels (Poly).vi"("error in (no error)"=w203, "input terminal"=w200, "instrument handle"=w204) -> ("error out"=w201:errorcluster, "instrument handle out"=w202:refnum<k15>)  [unwired: 7 in]
        n76 = property class="niDCPower"(reference=w202, error in=w201, "Measure When"=w228, "Aperture Time"=w205) -> (reference out=w226:refnum<k15>, error out=w227:errorcluster)
        n77 = call <instrlib>:"niDCPower Commit With Channels.vi"("error in (no error)"=w227, "channel name"=w174, "instrument handle"=w226) -> ("error out"=w216:errorcluster, "instrument handle out"=w218:refnum<k15>)  [unwired: 7 in]
        n78 = property class="niDCPower"(reference=w218, error in=w216, "Active Channel"=w174) -> (reference out=w217:refnum<k15>, error out=w211:errorcluster, "Measure Record dt"=w193:dbl)
        n79 = Bundle By Name(cluster=w213, "Measure record length smu"=w209, "Source out"=w217, "measurement results.dt"=w193) -> (w212:T3)
      }
      frame "ConfigureLoadToSinglepoint" {
        w259 = 1027 items=["Automatically after Source Complete"=1025, "On Demand"=1026, "On Measure Trigger"=1027] ("Measurement:Advanced:Measure When")
        w273 = T8 1007 items=["DC Voltage"=1006, "DC Current"=1007, "Pulse Voltage"=1049, "Pulse Current"=1050] ("output function")
        w272 = T5 1020 items=["Single Point"=1020, "Sequence"=1021] ("source mode")
        n80 = Unbundle By Name(w263) -> ("Load channel name"=w254:string, "Load out"=w279:refnum<k15>)
        n81 = Unbundle By Name(w267) -> ("Load transient response"=w246:i32, "Load current gain bandwidth"=w249:dbl, "Load current compensation frequency"=w248:dbl, "Load current pole-zero ratio"=w247:dbl)
        n82 = Unbundle By Name(w263) -> ("Measure record length smu"=w266:i32, "Aperture time"=w265:dbl)
        n83 = Unbundle By Name(w263) -> ("Source terminal name"=w278:string, "Measure load and scope terminal name"=w277:string)
        n84 = call <instrlib>:"niDCPower Configure Source Mode With Channels.vi"("error in (no error)"=w268, "source mode"=w272, "channel name"=w254, "instrument handle"=w279) -> ("error out"=w270:errorcluster, "instrument handle out"=w271:refnum<k15>)  [unwired: 6 in]
        n85 = call <instrlib>:"niDCPower Configure Output Function.vi"("error in (no error)"=w270, "output function"=w273, "channel name"=w254, "instrument handle"=w271) -> ("error out"=w275:errorcluster, "instrument handle out"=w274:refnum<k15>)  [unwired: 6 out]
        n86 = call-poly <instrlib>:"niDCPower Configure Trigger With Channels (Poly).vi"("error in (no error)"=w275, "input terminal"=w278, "channel name"=w254, "instrument handle"=w274) -> ("error out"=w269:errorcluster, "instrument handle out"=w276:refnum<k15>)  [unwired: 6 in]
        n87 = property class="niDCPower"(reference=w276, error in=w269, "Transient Response"=w246, "Measure Record Length"=w266, "Aperture Time"=w265) -> (reference out=w253:refnum<k15>, error out=w252:errorcluster)
        n88 = case shown="Default" w246 {
          tunnel: w253 -> [w281 w288]
          tunnel: w252 -> [w280 w287]
          tunnel: [w281 w286] -> w251
          tunnel: [w280 w285] -> w250
          tunnel: w249 -> [_ w284]
          tunnel: w248 -> [_ w283]
          tunnel: w247 -> [_ w282]
          frame Default {
          }
          frame 1042 {
            n89 = property class="niDCPower"(reference=w288, error in=w287, "Current GBW"=w284, "Current Compensation Freq"=w283, "Current Pole-Zero Ratio"=w282) -> (reference out=w286:refnum<k15>, error out=w285:errorcluster)
          }
        }
        n90 = call-poly <instrlib>:"niDCPower Configure Trigger With Channels (Poly).vi"("error in (no error)"=w250, "input terminal"=w277, "channel name"=w254, "instrument handle"=w251) -> ("error out"=w258:errorcluster, "instrument handle out"=w256:refnum<k15>)  [unwired: 6 in]
        n91 = property class="niDCPower"(reference=w256, error in=w258, "Measure When"=w259) -> (reference out=w255:refnum<k15>, error out=w257:errorcluster)
        n92 = call <instrlib>:"niDCPower Commit With Channels.vi"("error in (no error)"=w257, "channel name"=w254, "instrument handle"=w255) -> ("error out"=w264:errorcluster, "instrument handle out"=w262:refnum<k15>)  [unwired: 7 in]
        n93 = Bundle By Name(cluster=w263, "Load out"=w262) -> (w261:T3)
      }
      frame "StartSourceLoad" {
        n94 = Unbundle By Name(w292) -> ("Source out"=w294:refnum<k15>, "Source channel name"=w295:string, "Load out"=w298:refnum<k15>, "Load channel name"=w299:string)
        n95 = flat-sequence {
          tunnel: [w311] -> w303
          tunnel: [w310] -> w302
          tunnel: [w309] -> w301
          tunnel: w298 -> [w308]
          tunnel: w294 -> [w307]
          tunnel: w295 -> [w304]
          tunnel: w299 -> [w305]
          tunnel: [w304] -> w300
          tunnel: w293 -> [w306]
          tunnel: w303 -> [w318]
          tunnel: w302 -> [w317]
          tunnel: w301 -> [w314]
          tunnel: [w315] -> w296
          tunnel: [w316] -> w290
          tunnel: [w314] -> w297
          tunnel: w300 -> [w313]
          frame #0 {
            n96 = call <instrlib>:"niDCPower Initiate With Channels.vi"("error in (no error)"=w306, "channel name"=w305, "instrument handle"=w308) -> ("error out"=w312:errorcluster, "instrument handle out"=w309:refnum<k15>)  [unwired: 7 in]
            n97 = call <instrlib>:"niDCPower Initiate With Channels.vi"("error in (no error)"=w312, "channel name"=w304, "instrument handle"=w307) -> ("error out"=w310:errorcluster, "instrument handle out"=w311:refnum<k15>)  [unwired: 7 in]
          }
          frame #1 {
            w319 = T4 1033 items=["Source Complete Event"=1030, "Measure Complete Event"=1031, "Sequence Iteration Complete Event"=1032, "Sequence Engine Done Event"=1033] ("event")
            n98 = call <instrlib>:"niDCPower Wait For Event With Channels.vi"("error in (no error)"=w317, "event"=w319, "channel name"=w313, "instrument handle"=w318) -> ("error out"=w316:errorcluster, "instrument handle out"=w315:refnum<k15>)  [unwired: 6 in]
          }
        }
        n99 = Bundle By Name(cluster=w292, "Source out"=w296, "Load out"=w297) -> (w291:T3)
      }
      frame "StartSourceLoadAndScope" {
        n100 = Unbundle By Name(w329) -> ("Source out"=w333:refnum<k15>, "Source channel name"=w332:string, "Load out"=w322:refnum<k15>, "Load channel name"=w321:string, "Scope out"=w327:refnum<k15>)
        n101 = flat-sequence {
          tunnel: [w348] -> w337
          tunnel: [w347] -> w336
          tunnel: [w346] -> w335
          tunnel: w322 -> [w345]
          tunnel: w333 -> [w344]
          tunnel: w332 -> [w338]
          tunnel: w321 -> [w339]
          tunnel: [w338] -> w334
          tunnel: w328 -> [w343]
          tunnel: w327 -> [w341]
          tunnel: [w340] -> w326
          tunnel: w337 -> [w356]
          tunnel: w336 -> [w355]
          tunnel: w335 -> [w352]
          tunnel: [w353] -> w331
          tunnel: [w354] -> w324
          tunnel: [w352] -> w330
          tunnel: w334 -> [w351]
          tunnel: [w350] -> w325
          tunnel: w326 -> [w350]
          frame #0 {
            n102 = call <instrlib>:"niScope Initiate Acquisition.vi"("instrument handle"=w341, "error in"=w343) -> ("instrument handle out"=w340:refnum<k15>, "error out"=w342:errorcluster)  [unwired: 12 in]
            n103 = call <instrlib>:"niDCPower Initiate With Channels.vi"("error in (no error)"=w342, "channel name"=w339, "instrument handle"=w345) -> ("error out"=w349:errorcluster, "instrument handle out"=w346:refnum<k15>)  [unwired: 7 in]
            n104 = call <instrlib>:"niDCPower Initiate With Channels.vi"("error in (no error)"=w349, "channel name"=w338, "instrument handle"=w344) -> ("error out"=w347:errorcluster, "instrument handle out"=w348:refnum<k15>)  [unwired: 7 in]
          }
          frame #1 {
            w357 = T4 1033 items=["Source Complete Event"=1030, "Measure Complete Event"=1031, "Sequence Iteration Complete Event"=1032, "Sequence Engine Done Event"=1033] ("event")
            n105 = call <instrlib>:"niDCPower Wait For Event With Channels.vi"("error in (no error)"=w355, "event"=w357, "channel name"=w351, "instrument handle"=w356) -> ("error out"=w354:errorcluster, "instrument handle out"=w353:refnum<k15>)  [unwired: 6 in]
          }
        }
        n106 = Bundle By Name(cluster=w329, "Source out"=w331, "Load out"=w330, "Scope out"=w325) -> (w323:T3)
      }
      frame "PerformMeasurement" {
        n107 = Unbundle By Name(w377) -> ("Scope enable/disable"=w363:bool)
        n108 = Unbundle By Name(w381) -> ("Source out"=w373:refnum<k15>, "Source channel name"=w372:string, "Load out"=w375:refnum<k15>, "Load channel name"=w374:string, "Measure record length smu"=w370:i32)
        n109 = Unbundle By Name(w381) -> ("Scope out"=w369:refnum<k15>, "Scope channel name"=w368:string, "Measure record length scope"=w364:i32)
        n110 = call <instrlib>:"niDCPower Fetch Multiple.vi"("instrument handle"=w373, "channel name"=w372, "count (1)"=w370, "error in (no error)"=w382) -> ("instrument handle out"=w367:refnum<k15>, "voltage measurements"=w362:dbl[], "error out"=w376:errorcluster)  [unwired: 1 in, 8 out]
        n111 = call <instrlib>:"niDCPower Fetch Multiple.vi"("instrument handle"=w375, "channel name"=w374, "count (1)"=w370, "error in (no error)"=w376) -> ("instrument handle out"=w366:refnum<k15>, "voltage measurements"=w360:dbl[], "error out"=w371:errorcluster)  [unwired: 1 in, 8 out]
        n112 = case shown="True" w363 {
          tunnel: [w384 w391] -> w379
          tunnel: w371 -> [w384 w390]
          tunnel: w369 -> [w383 w389]
          tunnel: w368 -> [_ w388]
          tunnel: [w383 w387] -> w365
          tunnel: w364 -> [_ w386]
          tunnel: [_ w385] -> w361
          frame False {
          }
          frame True {
            n113 = call-poly <instrlib>:"niScope Fetch (poly).vi"("error in"=w390, "numSamples"=w386, "channels"=w388, "instrument handle"=w389) -> ("error out"=w391:errorcluster, "wfm"=w385:dbl[], "instrument handle out"=w387:refnum<k15>)  [unwired: 4 in, 1 out]
          }
        }
        n114 = Array Max & Min(array=w360) -> (max value=w359:dbl, min value=w358:dbl)  [unwired: 2 out]
        n115 = Bundle By Name(cluster=w381, "Source out"=w367, "measurement results.Source voltages"=w362, "Load out"=w366, "Scope out"=w365, "measurement results.Load voltages"=w360, "measurement results.Overshoot load voltage"=w359, "measurement results.Undershoot load voltage"=w358, "measurement results.Scope amplitudes"=w361) -> (w380:T3)
      }
      frame "Exit", Default {
        n116 = Unbundle By Name(w404) -> ("Scope enable/disable"=w392:bool)
        n117 = Unbundle By Name(w405) -> ("Source out"=w393:refnum<k15>, "Source channel name"=w394:string, "Load out"=w396:refnum<k15>, "Load channel name"=w395:string, "Scope out"=w397:refnum<k15>)
        n118 = case shown="True" w392 {
          tunnel: w409 -> [w410 w413]
          tunnel: [w410 w412] -> w398
          tunnel: w397 -> [_ w411]
          frame False {
          }
          frame True {
            n119 = call <instrlib>:"niScope Close.vi"("instrument handle"=w411, "error in"=w413) -> ("error out"=w412:errorcluster)  [unwired: 13 in]
          }
        }
        n120 = call <instrlib>:"niDCPower Abort With Channels.vi"("error in (no error)"=w398, "channel name"=w395, "instrument handle"=w396) -> ("error out"=w403:errorcluster, "instrument handle out"=w402:refnum<k15>)  [unwired: 7 in]
        n121 = call <instrlib>:"niDCPower Close.vi"("error in (no error)"=w403, "instrument handle"=w402) -> ("error out"=w399:errorcluster)  [unwired: 9 in]
        n122 = call <instrlib>:"niDCPower Abort With Channels.vi"("error in (no error)"=w399, "channel name"=w394, "instrument handle"=w393) -> ("error out"=w401:errorcluster, "instrument handle out"=w400:refnum<k15>)  [unwired: 7 in]
        n123 = call <instrlib>:"niDCPower Close.vi"("error in (no error)"=w401, "instrument handle"=w400) -> ("error out"=w408:errorcluster)  [unwired: 9 in]
      }
    }
  }
  "error out" <- w8
  "measure call context out" <- w5
  n124 = Unbundle By Name(w7) -> ("measurement results"=→"measurement results":T2)
